vi "Valid Folder Name.vi"(0 "Package":string, 11 "error in (no error)":errorcluster) -> (4 "Valid Package Name":string, 15 "error out":errorcluster)   [LabVIEW 2021, in "Measurement Builder.lvlib"]
uses:
  Measurement Builder.lvlib
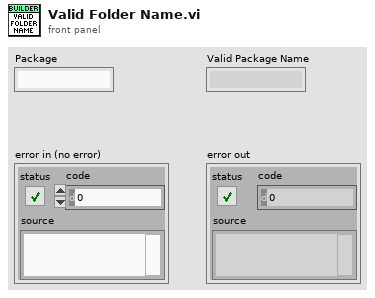
[diagram p1: front panel]
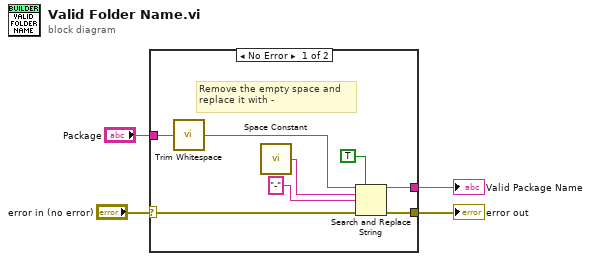
[diagram p0: block diagram]
diagram:
  n1 = case shown="No Error" "error in (no error)" {
    selector: "error in (no error)" -> [w12 w13]
    tunnel: [w11 w13] -> w3
    tunnel: [w10 _] -> w2
    tunnel: "Package" -> [w9 _]
    frame No Error {
      # "Remove the empty space and\nreplace it with -"
      n2 = call <vilib>:"Trim Whitespace.vi"("string"=w9) -> ("trimmed string"=w5:string)  [unwired: 1 in]
      n3 = call <vilib>:"Space Constant.vi"() -> ("String"=w6:string)
      n4 = Search and Replace String(replace all?=TRUE ("replace all? (F)"), input string=w5, search string=w6, replace string="-" ("replace string (\"\")"), error in=w12) -> (result string=w10:string, error out=w11:errorcluster)  [unwired: 3 in, 2 out]
    }
    frame Error {
    }
  }
  "error out" <- w3
  "Valid Package Name" <- w2
